vi "Set Velocity.vi"(8 "error in (no error)":errorcluster, 10 "Velocity In(deg/s)":dbl, 11 "SGDV_Ctrl_Class in":refnum<class "SGDV Motor.lvclass">) -> (0 "error out":errorcluster, 3 "SGDV_Ctrl_Class out":refnum<class "SGDV Motor.lvclass">)   [LabVIEW 2013, in "SGDV_Ctrl_v13_lib.lvlib" / "SGDV Motor.lvclass"]
uses:
  SGDV Motor.lvclass
  SGDV Motor.lvclass/SGDV Motor.ctl
  SGDV_Ctrl_v13_lib.lvlib
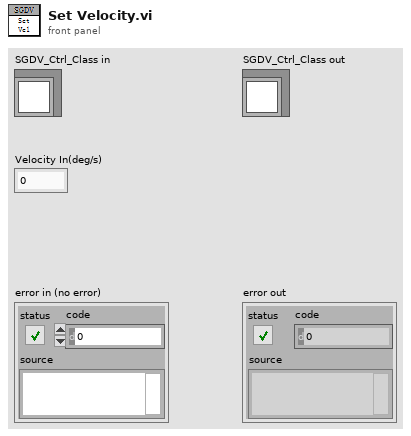
[diagram p1: front panel]
types:
  T1 = typedef "SGDV_Ctrl_v13_lib.lvlib/Motor Coefficients.ctl" = cluster{"Vel-Coefficient":dbl, "Enc-Coefficient":dbl, "Reduction-Ratio":dbl}
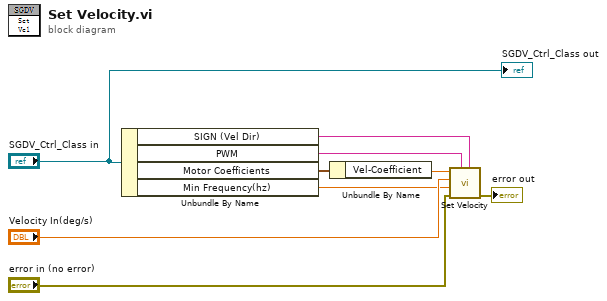
[diagram p0: block diagram]
diagram:
  n1 = Unbundle By Name("SGDV_Ctrl_Class in") -> ("SIGN (Vel Dir)"=w1:tag, "PWM"=w2:tag, "Motor Coefficients"=w8:T1, "Min Frequency(hz)"=w5:dbl)
  n2 = Unbundle By Name(w8) -> ("Vel-Coefficient"=w7:dbl)
  n3 = call "Set Velocity.vi"("SIGN (Vel Dir)"=w1, "PWM Channel Name"=w2, "error in (no error)"="error in (no error)", "Min Frequency(hz)"=w5, "Velocity In(deg/s)"="Velocity In(deg/s)", "Vel-Coefficient"=w7) -> ("error out"=→"error out":errorcluster)  [unwired: 5 in]
  "SGDV_Ctrl_Class out" <- "SGDV_Ctrl_Class in"
